vi "Area de un triangulo.vi"() -> ()   [LabVIEW 2021]
panel:
  out "?":string
  out "?":string
  in  "Base":dbl
  out "Area":dbl
  in  "Altura":dbl
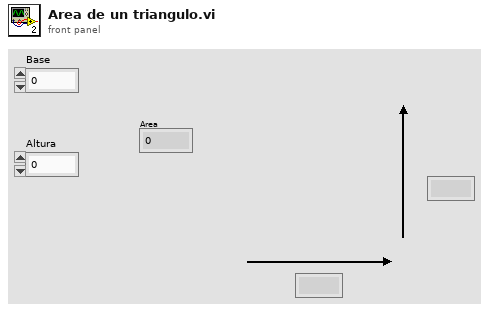
[diagram p1: front panel]
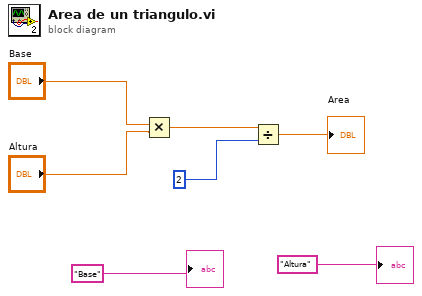
[diagram p0: block diagram]
diagram:
  n1 = Multiply(x="Base", y="Altura") -> (x*y=w5:dbl)
  n2 = Divide(x=w5, y=2) -> (x/y=→"Area":dbl)
  "?" <- "Altura"
  "?" <- "Base"
